vi "simplePath.vi"() -> ()   [LabVIEW 2018]
uses:
  <vilib>/Model Interface Toolkit/Model Interface Toolkit.lvclass/Model Interface Toolkit.ctl
  <vilib>/Model Interface Toolkit/Model Update.vi
  <vilib>/Model Interface Toolkit/Tick Model.vi
  <vilib>/Model Interface Toolkit/Probe Signals.vi
  <vilib>/Model Interface Toolkit/Multirate/Dispatch Model Tasks.vi
  <vilib>/Model Interface Toolkit/Call Model Start Routine.vi
  <vilib>/Model Interface Toolkit/Handle Error.vi
  <vilib>/Model Interface Toolkit/Multirate/Wait on Tasks.vi
  GlobalVariables.vi
  <vilib>/Model Interface Toolkit/Check Error.vi
  <vilib>/Model Interface Toolkit/Generate Error Cluster.vi
  <vilib>/Platform/TimedLoop/scheduler/LVUserAPI/Fire Software-Triggered Timing Source.vi
  <vilib>/addons/control/pid/pid.llb/PID (DBL).vi
  <vilib>/Model Interface Toolkit/Model Interface Toolkit.lvclass
  <vilib>/addons/control/pid/NI_PID_pid.lvlib
panel:
  out "steerAngle 2":dbl
  in  "D 2":dbl=0.01
  in  "I 2":dbl
  in  "P 2":dbl=70.0
  in  "missionFlag":u8=2
  in  "preDist":dbl=7.0
  out "路径":path
  out "lon":dbl format="%#.11g"
  out "lat":dbl format="%#.11g"
  out "steerAngle":dbl
  out "offset":dbl
  in  "D":dbl=0.3
  in  "I":dbl
  in  "P":dbl=46.0
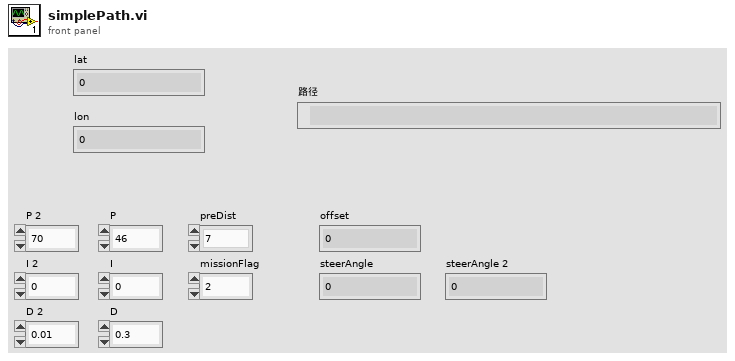
[diagram p1: front panel]
types:
  T1 = cluster{"Name":string, "port":string, "sequence":string, "idleTime":string, "timeStatus":string, "week":string, "seconds":string, "receiverStatus":string, "reserved":string, "receiverVersion":string, "insStatus":string, "posType":string, "lat":string, "lon":string, "height":string, "undulation":string, "northVel":string, "eastVel":string, "upVel":string, "roll":string, "pitch":string, "azimuth":string, "latStandardDevivation":string, "lonStandardDevivation":string, "heightStandardDevivation":string, "northStandardDevivation":string, "eastStandardDevivation":string, "upStandardDevivation":string, "rollStandardDevivation":string, "pitchStandardDevivation":string, "azimuthStandardDevivation":string, "extSolSat":string, "timeSinceUpdate":string, "CRC":string, "#INSPVAXA":string}
  T2 = cluster{"EMS+ECS+EPS Enable":bool, "HAD_Angle_Wheel":dbl, "HAD_Anglular_Velocity":dbl}
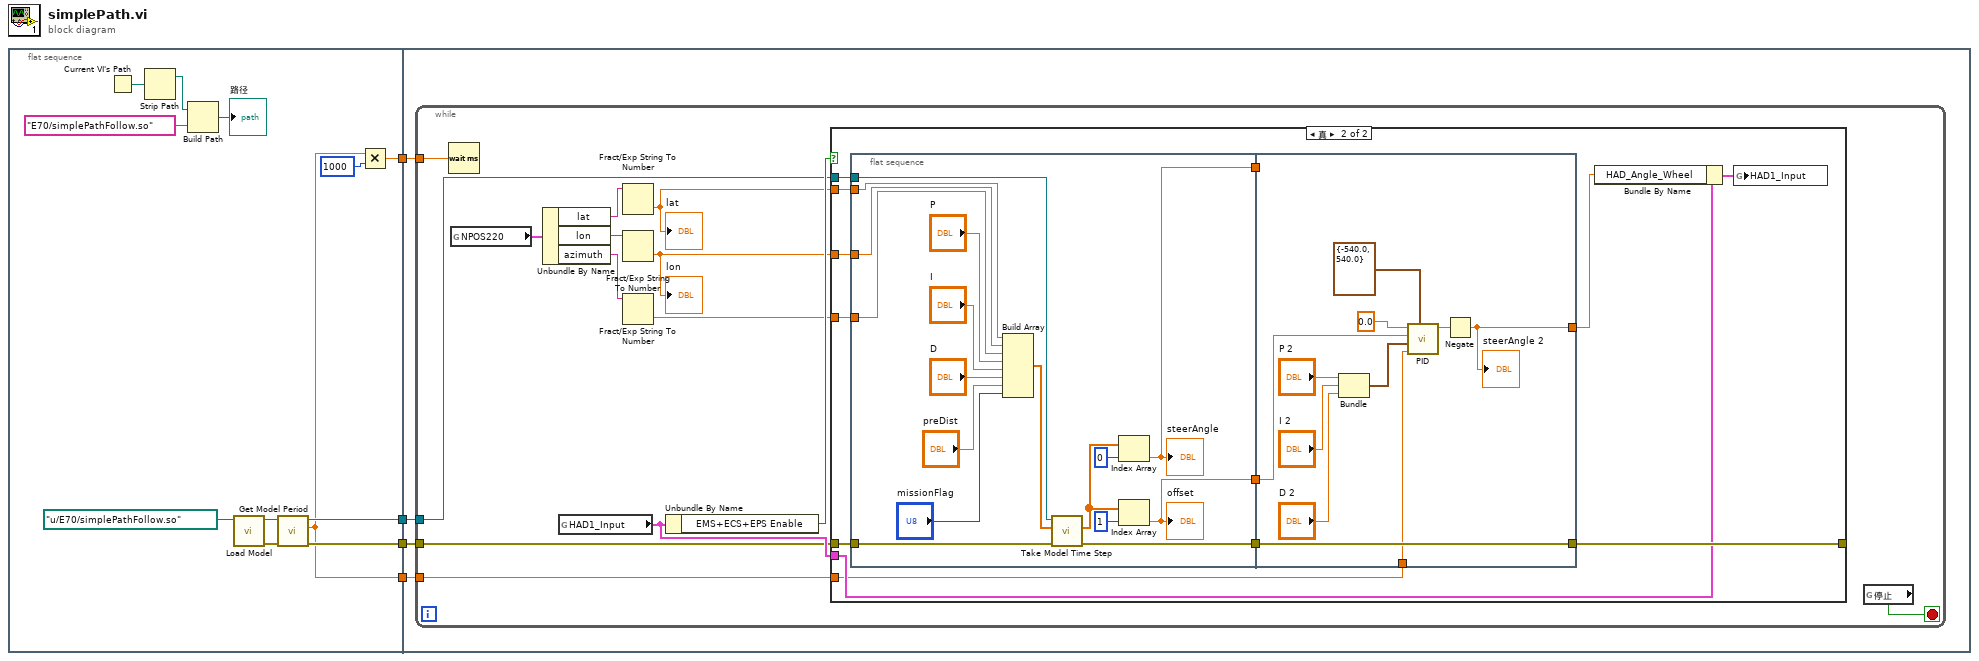
[diagram p0: block diagram]
diagram:
  n1 = flat-sequence {
    tunnel: [w9] -> w4
    tunnel: [w10] -> w3
    tunnel: [w7] -> w2
    tunnel: [w5] -> w1
    tunnel: w4 -> [w19]
    tunnel: w3 -> [w20]
    tunnel: w2 -> [w18]
    tunnel: w1 -> [w17]
    frame #0 {
      n2 = Current VI's Path() -> (path=w15:path)
      n3 = Strip Path(path=w15) -> (stripped path=w14:path)  [unwired: 1 out]
      n4 = Build Path(base path=w14, name or relative path="E70/simplePathFollow.so") -> (appended path=→"路径":path)
      n5 = call <vilib>:"Load Model.vi"("Model Path"=path "u:/E70/simplePathFollow.so") -> ("error out"=w11:errorcluster, "Model out"=w12:refnum<class "Model Interface Toolkit.lvclass">)  [unwired: 9 in]
      n6 = call <vilib>:"Get Model Period.vi"("error in"=w11, "Model in"=w12) -> ("error out"=w10:errorcluster, "Model Period (s)"=w5:dbl, "Model out"=w9:refnum<class "Model Interface Toolkit.lvclass">)  [unwired: 7 in]
      n7 = Multiply(x=w5, y=1000) -> (x*y=w7:dbl)
    }
    frame #1 {
      n8 = while {
        tunnel: w20 -> [w31]
        tunnel: w19 -> [w30]
        tunnel: w18 -> [w29]
        tunnel: w17 -> [w21]
        stop <- w34 stop-if-true
        n9 = Wait (ms)(milliseconds to wait=w29) -> ()  [unwired: 1 out]
        n10 = global read "GlobalVariables.vi" "NPOS220"() -> (w28:T1)
        n11 = Unbundle By Name(w28) -> ("lat"=w22:string, "lon"=w27:string, "azimuth"=w26:string)
        n12 = global read "GlobalVariables.vi" "HAD1_Input"() -> (w32:T2)
        n13 = Fract/Exp String To Number(string=w22) -> (number=w23:dbl)  [unwired: 3 in, 1 out]
        "lat" <- w23
        n14 = Fract/Exp String To Number(string=w27) -> (number=w24:dbl)  [unwired: 3 in, 1 out]
        "lon" <- w24
        n15 = Fract/Exp String To Number(string=w26) -> (number=w25:dbl)  [unwired: 3 in, 1 out]
        n16 = Unbundle By Name(w32) -> ("EMS+ECS+EPS Enable"=w33:bool)
        n17 = case shown="真" w33 {
          tunnel: w32 -> [_ w42]
          tunnel: w31 -> [w35 w48]
          tunnel: w30 -> [_ w47]
          tunnel: [w35 w46] -> _
          tunnel: w25 -> [_ w45]
          tunnel: w24 -> [_ w44]
          tunnel: w23 -> [_ w43]
          tunnel: w21 -> [_ w36]
          frame False {
          }
          frame True {
            n18 = flat-sequence {
              tunnel: w48 -> [w63]
              tunnel: w47 -> [w62]
              tunnel: w45 -> [w55]
              tunnel: w44 -> [w54]
              tunnel: w43 -> [w53]
              tunnel: [w61] -> w40
              tunnel: [w50] -> w39
              tunnel: [w49] -> w37
              tunnel: [w76] -> w46
              tunnel: w40 -> [w76]
              tunnel: w39 -> [_]
              tunnel: [w69] -> w38
              tunnel: w37 -> [w68]
              tunnel: w36 -> [w67]
              frame #0 {
                n19 = Build Array(w53, w54, w55, "P", "I", "D", "preDist", "missionFlag") -> (w59:dbl[])
                n20 = call <vilib>:"Take Model Time Step.vi"("error in (no error)"=w63, "Inport Array"=w59, "Model in"=w62) -> ("error out"=w61:errorcluster, "Outport Array out"=w60:dbl[])  [unwired: 6 in, 1 out]
                n21 = Index Array(array=w60, index=0) -> (element=w50:dbl)
                "steerAngle" <- w50
                n22 = Index Array(array=w60, index=1) -> (element=w49:dbl)
                "offset" <- w49
              }
              frame #1 {
                n23 = Bundle("P 2"="P 2", "I 2"="I 2", "D 2"="D 2") -> (w75:cluster{"P 2":dbl, "I 2":dbl, "D 2":dbl})  [unwired: 1 in]
                n24 = call-poly <vilib>:"PID.vi"("output range"=cluster{dbl, dbl} {-540.0, 540.0}, "dt (s)"=w67, "PID gains"=w75, "process variable"=w68, "setpoint"=0.0) -> ("output"=w73:dbl)  [unwired: 5 in, 1 out]
                n25 = Negate(x=w73) -> (-x=w69:dbl)
                "steerAngle 2" <- w69
              }
            }
            n26 = Bundle By Name(cluster=w42, "HAD_Angle_Wheel"=w38) -> (w41:T2)
            n27 = global write "GlobalVariables.vi" "HAD1_Input"(w41) -> ()
          }
        }
        n28 = global read "GlobalVariables.vi" "停止"() -> (w34:bool)
      }
    }
  }
